vi "Impedance_SingleStats.vi"() -> ()   [LabVIEW 2020]
uses:
  <vilib>/Analysis/NI_AALBase.lvlib
panel:
  out "output cluster":T1 {"Mean |Z|" format="%#_6p"; "standard deviation |Z|" format="%#_6p"; "Mean Phase" format="%#_6p"; "standard deviation Phase" format="%#_6p"; "mean Ls" format="%#_6p"; "Standard dev. Ls" format="%#_6p"; "mean Real(Z)" format="%#_6p"; "Std. dev Real(Z)" format="%#_6p"; "mean Cs" format="%#_6p"; "Std. Dev. Cs" format="%#_6p"; "Mean Rp" format="%#_6p"; "Std. Dev. Rp" format="%#_6p"; "Mean Cp" format="%#_6p"; "Std. Dev. Cp" format="%#_6p"}
  out "standard deviation":dbl format="%.2p"
  out "Progress":i32(slide)=90 scale=0.0..100.0
  in  "Tab Control":enum32{"Input Params", "Output Plots"}(tab)
  in  "LCR Params":T2={"Rg_Vmon"=5000.0, "Rg_Imon"=5000.0, "ESL_Cal"=2.5e-07, "ESR_Cal"=0.0, "Cp_Cal"=0.0, "Rp_Cal"=1000000000.0, "UseCorrection"=FALSE, "R_Shunt"=100.0}
  in  "Test Params Cluster":T3={"Test Freq. (Hz)"=25000.0, "Output Signal Amplitude\nVolts Pk"=0.1, "Sampling Time (s)"=0.1, "Sampling Rate (Hz)"=2000000.0, "Output Channel"="PXI1Slot2/ao1", "Current Channel"="PXI1Slot2/ai1", "Voltage Channel"="PXI1Slot2/ai0", "Trigger Channel"="/PXI1Slot2/ao/StartTrigger", "Number of runs"=10} {"Sampling Rate (Hz)" format="%#_6p"}
  in  "Save Every\nRun File?":bool
  in  "samples":i32=10
  out "Test Number":i32=9
  in  "File Name String":string="TestStats"
  in  "Save Path":path=path "C:/Users/Human-MPI/Desktop/Temp"
  in  "Experiment Title":string="Experiment Title"
  in  "Save final stats":bool
  out "Phase Chart":dbl(graph)=95.45920483054104
  out "Real(Z) Chart":dbl(graph)=-0.005381459479146001
  out "Capacitance Chart":dbl(graph)=-0.00011305866221997783
  out "|Z| over time":dbl(graph)=0.05656537092200194
  out "Inductance Chart":dbl(graph)=3.584729613913086e-07
  out "Current Run Results":T4={"|Z|"=0.05656537092200194, "Phase(Z)"=95.45920483054104, "Re(Z)"=-0.005381459479146001, "Imag(Z)"=0.056308801100875626, "Ls"=3.584729613913086e-07, "Cs"=-0.00011305866221997783, "Rp"=-0.5945675517845621, "Cp"=-0.00011203536283595137} {"|Z|" format="%#_6p"; "Phase(Z)" format="%#_6p"; "Re(Z)" format="%#_6p"; "Imag(Z)" format="%#_6p"; "Ls" format="%#_6p"; "Cs" format="%#_6p"; "Rp" format="%#_6p"; "Cp" format="%#_6p"}
  out "Histogram Graph Phase":T5(graph)={"X Values"=[95.20701436407293, 95.2415389303248, 95.27606349657665, 95.31058806282851, 95.34511262908038, 95.37963719533224, 95.4141617615841, 95.44868632783596, 95.48321089408782, 95.51773546033968], "Histogram: h(x)"=[1, 0, 0, 2, 1, 1, 2, 1, 1, 1]}
  out "Histogram Graph Mag":T5(graph)={"X Values"=[0.05657083132191394, 0.05658175212173795, 0.05659267292156196, 0.05660359372138597, 0.05661451452120998, 0.05662543532103399, 0.056636356120858, 0.05664727692068201, 0.05665819772050602, 0.056669118520330033], "Histogram: h(x)"=[1, 0, 1, 0, 1, 0, 4, 1, 1, 1]}
  # "Will create as many files as there are number of runs\n(Not typical)"
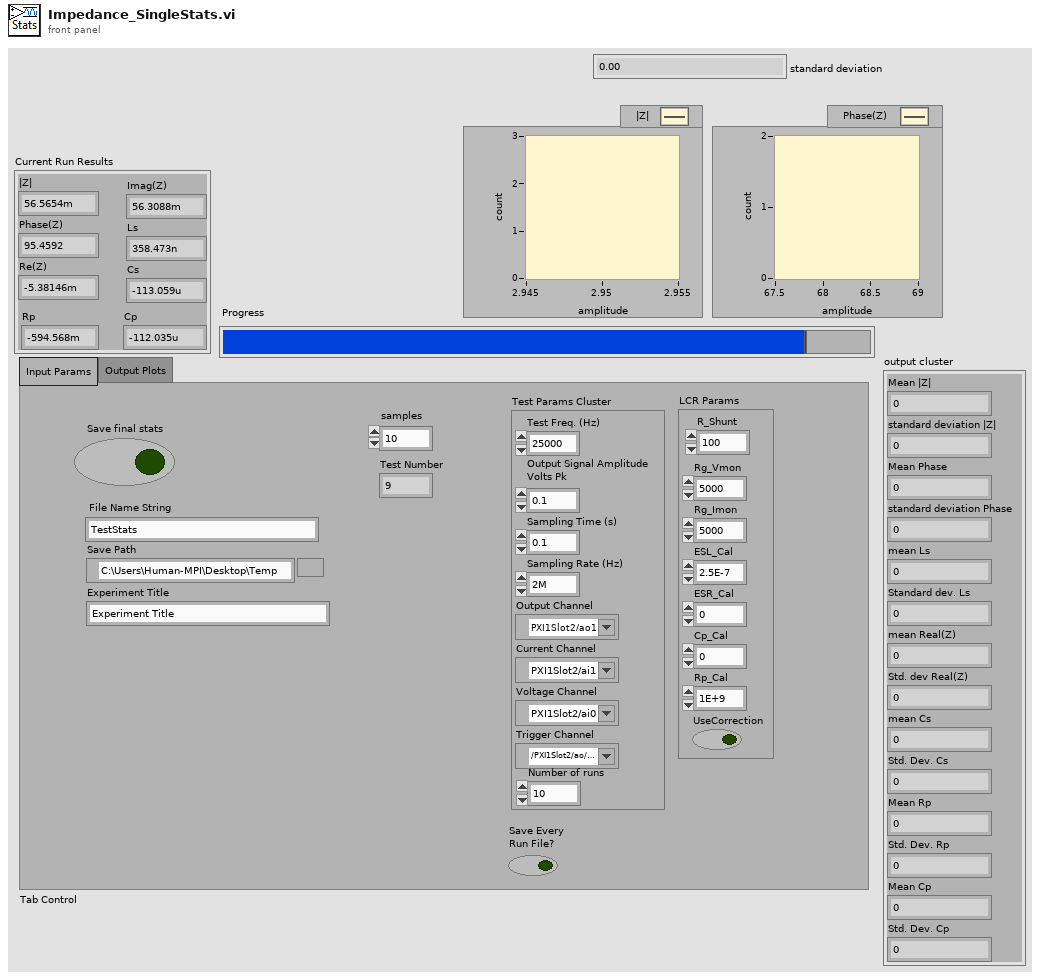
[diagram p1: front panel]
types:
  T1 = cluster{"Mean |Z|":dbl, "standard deviation |Z|":dbl, "Mean Phase":dbl, "standard deviation Phase":dbl, "mean Ls":dbl, "Standard dev. Ls":dbl, "mean Real(Z)":dbl, "Std. dev Real(Z)":dbl, "mean Cs":dbl, "Std. Dev. Cs":dbl, "Mean Rp":dbl, "Std. Dev. Rp":dbl, "Mean Cp":dbl, "Std. Dev. Cp":dbl}
  T2 = cluster{"Rg_Vmon":dbl, "Rg_Imon":dbl, "ESL_Cal":dbl, "ESR_Cal":dbl, "Cp_Cal":dbl, "Rp_Cal":dbl, "UseCorrection":bool, "R_Shunt":dbl}
  T3 = cluster{"Test Freq. (Hz)":dbl, "Output Signal Amplitude\nVolts Pk":dbl, "Sampling Time (s)":dbl, "Sampling Rate (Hz)":dbl, "Output Channel":tag, "Current Channel":tag, "Voltage Channel":tag, "Trigger Channel":tag, "Number of runs":i32}
  T4 = cluster{"|Z|":dbl, "Phase(Z)":dbl, "Re(Z)":dbl, "Imag(Z)":dbl, "Ls":dbl, "Cs":dbl, "Rp":dbl, "Cp":dbl}
  T5 = cluster{"X Values":dbl[], "Histogram: h(x)":i32[]}
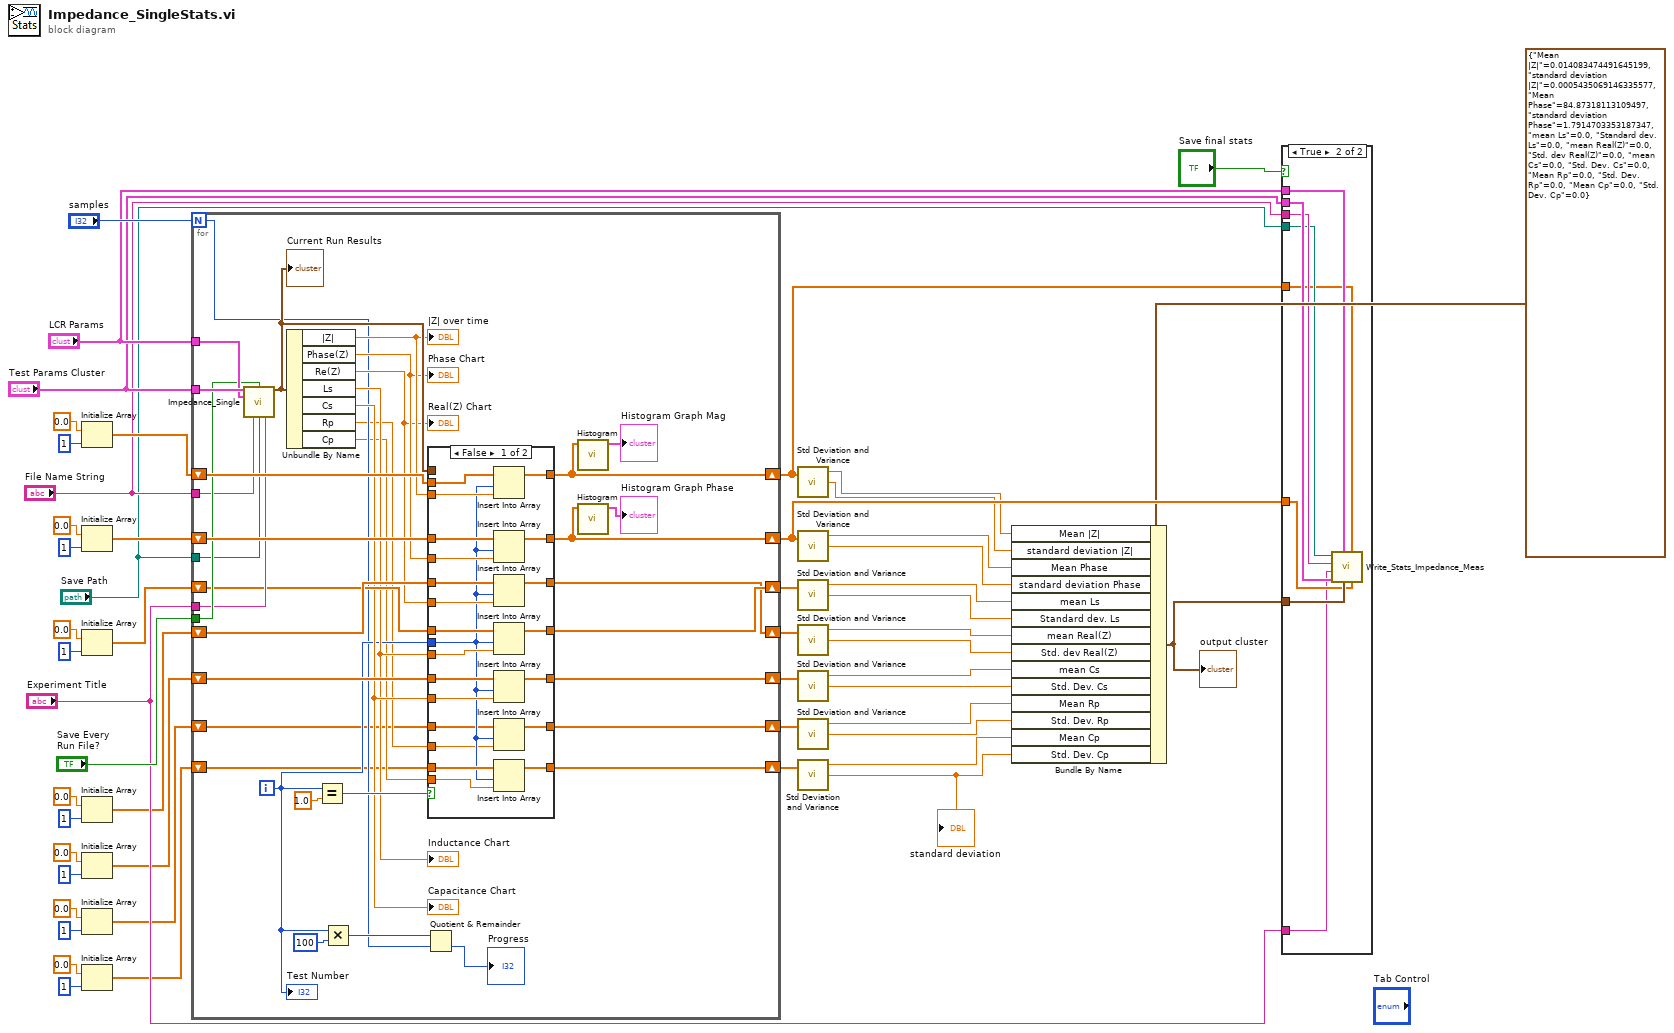
[diagram p0: block diagram]
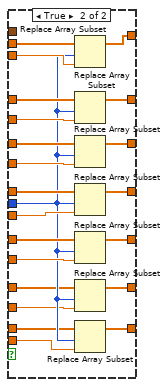
[diagram p2: hidden frame]
diagram:
  n1 = Initialize Array(0.0 ("element"), 1 ("dimension size")) -> (w51:dbl[])
  n2 = Initialize Array(0.0 ("element"), 1 ("dimension size")) -> (w49:dbl[])
  n3 = Initialize Array(0.0 ("element"), 1 ("dimension size")) -> (w25:dbl[])
  n4 = Initialize Array(0.0 ("element"), 1 ("dimension size")) -> (w26:dbl[])
  n5 = Initialize Array(0.0 ("element"), 1 ("dimension size")) -> (w24:dbl[])
  n6 = Initialize Array(0.0 ("element"), 1 ("dimension size")) -> (w9:dbl[])
  n7 = Initialize Array(0.0 ("element"), 1 ("dimension size")) -> (w8:dbl[])
  n8 = for {
    N: "samples" -> [w59]
    shift-right: [w82] -> w38
    shift-left: w51 -> [w89]
    shift-right: [w83] -> w39
    shift-left: w49 -> [w88]
    tunnel: "Test Params Cluster" -> [w81]
    tunnel: "LCR Params" -> [w80]
    tunnel: "Save Every\nRun File?" -> [w79]
    tunnel: "File Name String" -> [w78]
    tunnel: "Save Path" -> [w77]
    tunnel: "Experiment Title" -> [w76]
    shift-right: [w64] -> w21
    shift-left: w26 -> [w72]
    shift-right: [w65] -> w22
    shift-left: w25 -> [w71]
    shift-right: [w66] -> w23
    shift-left: w24 -> [w70]
    shift-right: [w53] -> w7
    shift-left: w9 -> [w56]
    shift-right: [w54] -> w6
    shift-left: w8 -> [w55]
    i -> [w60]
    n9 = call "Impedance_Single.vi"("Test Params Cluster"=w81, "SaveFile?"=w79, "LCR Params"=w80, "File Name String"=w78, "Path"=w77, "Experiment Title"=w76) -> ("Mean Signal\nImpedance cluster"=w75:T4)  [unwired: 9 in]
    "Current Run Results" <- w75
    n10 = Unbundle By Name(w75) -> ("|Z|"=w74:dbl, "Phase(Z)"=w73:dbl, "Re(Z)"=w67:dbl, "Ls"=w68:dbl, "Cs"=w69:dbl, "Rp"=w58:dbl, "Cp"=w57:dbl)
    "|Z| over time" <- w74
    "Real(Z) Chart" <- w67
    "Phase Chart" <- w73
    "Inductance Chart" <- w68
    "Capacitance Chart" <- w69
    n11 = Equal?(x=w60, y=1.0) -> (x = y?=w85:bool)
    n12 = Multiply(x=w60, y=100) -> (x*y=w61:i32)
    n13 = Quotient & Remainder(x=w61, y=w59) -> (floor(x/y)=→"Progress":i32)  [unwired: 1 out]
    n14 = case shown="False" w85 {
      tunnel: w89 -> [w111 w133]
      tunnel: w88 -> [w109 w132]
      tunnel: w60 -> [w94 w118]
      tunnel: [w108 w131] -> w83
      tunnel: [w110 w130] -> w82
      tunnel: w75 -> [_ _]
      tunnel: w74 -> [w106 w129]
      tunnel: w73 -> [w107 w128]
      tunnel: w72 -> [w104 w127]
      tunnel: w71 -> [w105 w126]
      tunnel: w70 -> [w103 w125]
      tunnel: w69 -> [w102 w124]
      tunnel: w68 -> [w101 w123]
      tunnel: w67 -> [w100 w122]
      tunnel: [w99 w121] -> w66
      tunnel: [w98 w120] -> w65
      tunnel: [w97 w119] -> w64
      tunnel: w58 -> [w91 w117]
      tunnel: w57 -> [w90 w116]
      tunnel: w56 -> [w93 w115]
      tunnel: w55 -> [w96 w114]
      tunnel: [w95 w113] -> w54
      tunnel: [w92 w112] -> w53
      frame False {
        n15 = Insert Into Array(array=w111, index=w94, new element=w106) -> (w110:dbl[])
        n16 = Insert Into Array(array=w109, index=w94, new element=w107) -> (w108:dbl[])
        n17 = Insert Into Array(array=w104, index=w94, new element=w100) -> (w97:dbl[])
        n18 = Insert Into Array(array=w105, index=w94, new element=w101) -> (w98:dbl[])
        n19 = Insert Into Array(array=w103, index=w94, new element=w102) -> (w99:dbl[])
        n20 = Insert Into Array(array=w93, index=w94, new element=w91) -> (w92:dbl[])
        n21 = Insert Into Array(array=w96, index=w94, new element=w90) -> (w95:dbl[])
      }
      frame True {
        n22 = Replace Array Subset(array=w133, new element=w129, index=w118) -> (w130:dbl[])
        n23 = Replace Array Subset(array=w132, new element=w128, index=w118) -> (w131:dbl[])
        n24 = Replace Array Subset(array=w127, new element=w122, index=w118) -> (w119:dbl[])
        n25 = Replace Array Subset(array=w126, new element=w123, index=w118) -> (w120:dbl[])
        n26 = Replace Array Subset(array=w125, new element=w124, index=w118) -> (w121:dbl[])
        n27 = Replace Array Subset(array=w115, new element=w117, index=w118) -> (w112:dbl[])
        n28 = Replace Array Subset(array=w114, new element=w116, index=w118) -> (w113:dbl[])
      }
    }
    n29 = call <vilib>:"Histogram.vi"("X"=w82) -> ("Histogram Graph"=→"Histogram Graph Mag":T5)  [unwired: 7 in, 3 out]
    n30 = call <vilib>:"Histogram.vi"("X"=w83) -> ("Histogram Graph"=→"Histogram Graph Phase":T5)  [unwired: 7 in, 3 out]
    "Test Number" <- w60
  }
  n31 = call <vilib>:"Std Deviation and Variance.vi"("X"=w38) -> ("mean"=w36:dbl, "standard deviation"=w35:dbl)  [unwired: 1 in, 1 out]
  n32 = call <vilib>:"Std Deviation and Variance.vi"("X"=w39) -> ("mean"=w34:dbl, "standard deviation"=w33:dbl)  [unwired: 1 in, 1 out]
  n33 = call <vilib>:"Std Deviation and Variance.vi"("X"=w22) -> ("mean"=w19:dbl, "standard deviation"=w18:dbl)  [unwired: 1 in, 1 out]
  n34 = call <vilib>:"Std Deviation and Variance.vi"("X"=w21) -> ("mean"=w17:dbl, "standard deviation"=w16:dbl)  [unwired: 1 in, 1 out]
  n35 = call <vilib>:"Std Deviation and Variance.vi"("X"=w23) -> ("mean"=w15:dbl, "standard deviation"=w14:dbl)  [unwired: 1 in, 1 out]
  n36 = call <vilib>:"Std Deviation and Variance.vi"("X"=w7) -> ("mean"=w5:dbl, "standard deviation"=w4:dbl)  [unwired: 1 in, 1 out]
  n37 = call <vilib>:"Std Deviation and Variance.vi"("X"=w6) -> ("mean"=w3:dbl, "standard deviation"=w2:dbl)  [unwired: 1 in, 1 out]
  "standard deviation" <- w2
  n38 = Bundle By Name(cluster=T1 {"Mean |Z|"=0.014083474491645199, "standard deviation |Z|"=0.0005435069146335577, "Mean Phase"=84.87318113109497, "standard deviation Phase"=1.7914703353187347, "mean Ls"=0.0, "Standard dev. Ls"=0.0, "mean Real(Z)"=0.0, "Std. dev Real(Z)"=0.0, "mean Cs"=0.0, "Std. Dev. Cs"=0.0, "Mean Rp"=0.0, "Std. Dev. Rp"=0.0, "Mean Cp"=0.0, "Std. Dev. Cp"=0.0} ("Output Stats Cluster"), "Mean |Z|"=w36, "standard deviation |Z|"=w35, "Mean Phase"=w34, "standard deviation Phase"=w33, "mean Ls"=w19, "Standard dev. Ls"=w18, "mean Real(Z)"=w17, "Std. dev Real(Z)"=w16, "mean Cs"=w15, "Std. Dev. Cs"=w14, "Mean Rp"=w5, "Std. Dev. Rp"=w4, "Mean Cp"=w3, "Std. Dev. Cp"=w2) -> (w1:T1)
  "output cluster" <- w1
  n39 = case shown="True" "Save final stats" {
    tunnel: w1 -> [_ w141]
    tunnel: w39 -> [_ w140]
    tunnel: "LCR Params" -> [_ w139]
    tunnel: "Test Params Cluster" -> [_ w138]
    tunnel: "Experiment Title" -> [_ w137]
    tunnel: "File Name String" -> [_ w136]
    tunnel: "Save Path" -> [_ w135]
    tunnel: w38 -> [_ w134]
    frame False {
    }
    frame True {
      n40 = call "Write_Stats_Impedance_Meas.vi"("Z Phase"=w140, "|Z| Mag"=w134, "Output Stats Cluster"=w141, "Compensation and Gain"=w139, "Test Params Cluster"=w138, "Experiment Title"=w137, "File Name String"=w136, "Path"=w135) -> ()  [unwired: 4 in]
    }
  }
